vi "RS485WriteRead.vi"(8 "error in (no error)":errorcluster, 10 "Control Option":T1(ring)=enum."SetLock", 11 "VISA resource name":refnum<visa-resource-name>="COM4") -> (0 "error out":errorcluster, 2 "Result":string, 3 "VISA resource name out":refnum<visa-resource-name>)   [LabVIEW 2016]
uses:
  <vilib>/Instr/_visa.llb/VISA Configure Serial Port (Instr).vi
panel:
  in  "flow control":u16(ring) items=["None"=0, "XON/XOFF"=1, "RTS/CTS"=2, "DTR/DSR"=4]
  in  "stop bits":u16(ring)=10 items=["1"=10, "1.5"=15, "2.0"=20]
  in  "parity":u16(ring)=2 items=["None", "Odd", "Even", "Mark", "Space"]
  in  "data bits":u16=8 min=5 max=8 step=1
  in  "baud rate":u32=1500000
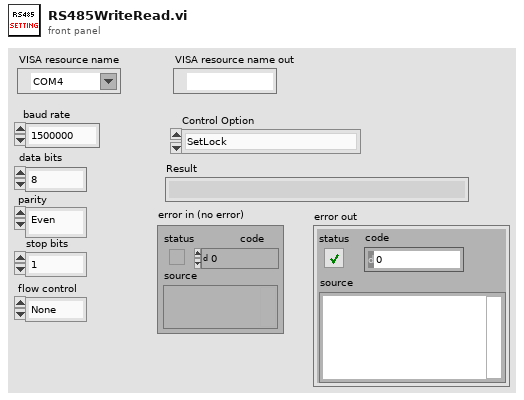
[diagram p1: front panel]
types:
  T1 = enum16{"ReadStream", "SetLock", "UnSetLock", "Read", "SetStreamMode", "UnSetStreammingMode"}
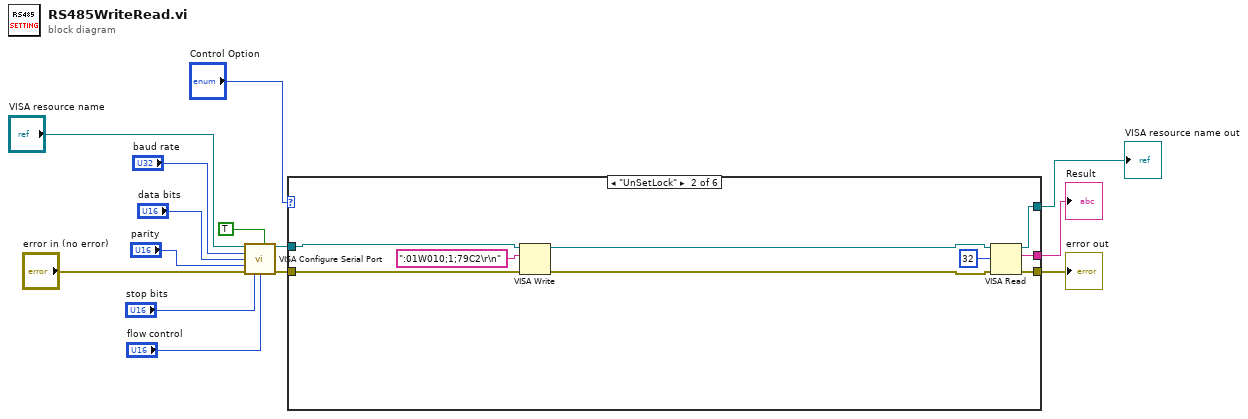
[diagram p0: block diagram]
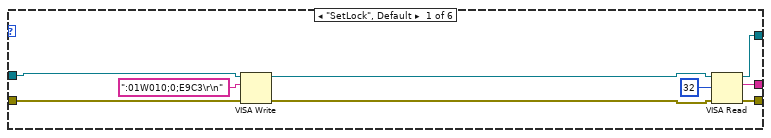
[diagram p2: hidden frame]
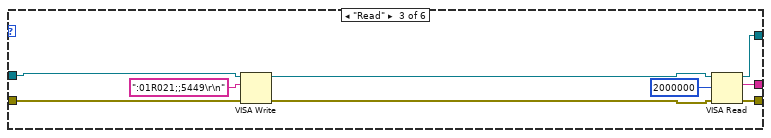
[diagram p3: hidden frame]
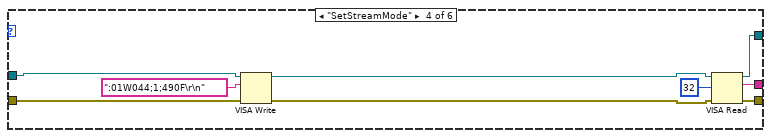
[diagram p4: hidden frame]
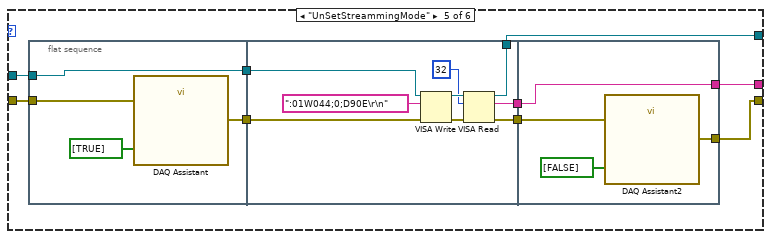
[diagram p5: hidden frame]
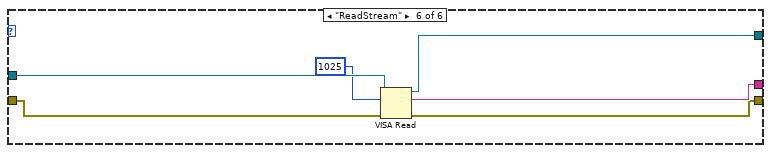
[diagram p6: hidden frame]
diagram:
  n1 = call-poly "VISA Configure Serial Port"("VISA resource name"="VISA resource name", "Enable Termination\nChar (T)"=TRUE, "baud rate (9600)"="baud rate", "data bits (8)"="data bits", "parity (0:none)"="parity", "error in (no error)"="error in (no error)", "stop bits (10: 1 bit)"="stop bits", "flow control (0:none)"="flow control") -> ("VISA resource name out"=w3:refnum<visa-resource-name>, "error out"=w7:errorcluster)  [unwired: 6 in]
  n2 = case shown="\"UnSetLock\"" "Control Option" {
    tunnel: [w19 w31 w36 w50 w52 w79] -> w8
    tunnel: w3 -> [w18 w29 w40 w48 w56 w82]
    tunnel: w7 -> [w17 w28 w41 w47 w57 w81]
    tunnel: [w16 w26 w34 w43 w58 w78] -> w5
    tunnel: [w15 w25 w33 w42 w51 w80] -> w1
    frame "SetLock", Default {
      n3 = VISA Write(VISA resource name=w18, write buffer=":01W010;0;E9C3\r\n", error in (no error)=w17) -> (VISA resource name out=w21:refnum<visa-resource-name>, error out=w20:errorcluster)  [unwired: 1 out]
      n4 = VISA Read(VISA resource name=w21, byte count=u32 32, error in (no error)=w20) -> (VISA resource name out=w15:refnum<visa-resource-name>, read buffer=w19:string, error out=w16:errorcluster)  [unwired: 1 out]
    }
    frame "UnSetLock" {
      n5 = VISA Write(VISA resource name=w29, write buffer=":01W010;1;79C2\r\n", error in (no error)=w28) -> (VISA resource name out=w30:refnum<visa-resource-name>, error out=w24:errorcluster)  [unwired: 1 out]
      n6 = VISA Read(VISA resource name=w30, byte count=u32 32, error in (no error)=w24) -> (VISA resource name out=w25:refnum<visa-resource-name>, read buffer=w31:string, error out=w26:errorcluster)  [unwired: 1 out]
    }
    frame "Read" {
      n7 = VISA Write(VISA resource name=w40, write buffer=":01R021;;5449\r\n" ("Command"), error in (no error)=w41) -> (VISA resource name out=w38:refnum<visa-resource-name>, error out=w37:errorcluster)  [unwired: 1 out]
      n8 = VISA Read(VISA resource name=w38, byte count=u32 2000000, error in (no error)=w37) -> (VISA resource name out=w33:refnum<visa-resource-name>, read buffer=w36:string, error out=w34:errorcluster)  [unwired: 1 out]
    }
    frame "SetStreamMode" {
      n9 = VISA Write(VISA resource name=w48, write buffer=":01W044;1;490F\r\n", error in (no error)=w47) -> (VISA resource name out=w49:refnum<visa-resource-name>, error out=w45:errorcluster)  [unwired: 1 out]
      n10 = VISA Read(VISA resource name=w49, byte count=u32 32, error in (no error)=w45) -> (VISA resource name out=w42:refnum<visa-resource-name>, read buffer=w50:string, error out=w43:errorcluster)  [unwired: 1 out]
    }
    frame "UnSetStreammingMode" {
      n11 = flat-sequence {
        tunnel: w57 -> [w62]
        tunnel: w56 -> [w61]
        tunnel: [w61] -> w55
        tunnel: [w60] -> w54
        tunnel: [w68] -> w59
        tunnel: w55 -> [w67]
        tunnel: w54 -> [w66]
        tunnel: [w65] -> w53
        tunnel: [w64] -> w51
        tunnel: w59 -> [w75]
        tunnel: [w74] -> w58
        tunnel: w53 -> [w73]
        tunnel: [w73] -> w52
        frame #0 {
          n12 = call "DAQ Assistant"("data"=bool[] [TRUE], "error in"=w62) -> ("error out"=w60:errorcluster)  [unwired: 16 in, 1 out]
        }
        frame #1 {
          n13 = VISA Write(VISA resource name=w67, write buffer=":01W044;0;D90E\r\n", error in (no error)=w66) -> (VISA resource name out=w70:refnum<visa-resource-name>, error out=w71:errorcluster)  [unwired: 1 out]
          n14 = VISA Read(VISA resource name=w70, byte count=u32 32, error in (no error)=w71) -> (VISA resource name out=w64:refnum<visa-resource-name>, read buffer=w65:string, error out=w68:errorcluster)  [unwired: 1 out]
        }
        frame #2 {
          n15 = call "DAQ Assistant2"("data"=bool[] [FALSE], "error in"=w75) -> ("error out"=w74:errorcluster)  [unwired: 16 in, 1 out]
        }
      }
    }
    frame "ReadStream" {
      n16 = VISA Read(VISA resource name=w82, byte count=1025, error in (no error)=w81) -> (VISA resource name out=w80:refnum<visa-resource-name>, read buffer=w79:string, error out=w78:errorcluster)  [unwired: 1 out]
    }
  }
  "Result" <- w8
  "error out" <- w5
  "VISA resource name out" <- w1
